vi "GetDeviceDetails.vi"(0 "reference in":refnum<class "Driver_Template.lvclass">, 11 "error in (no error)":errorcluster) -> (4 "reference out":refnum<class "Driver_Template.lvclass">, 6 "Name":string, 8 "Model":string, 10 "FW_Version":string, 13 "Is Device?":bool, 14 "SN":string, 15 "error out":errorcluster)   [LabVIEW 2014]
uses:
  Driver_Template.lvclass
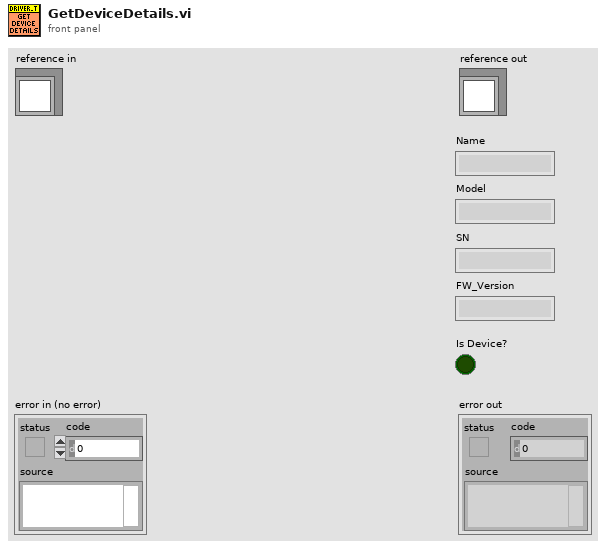
[diagram p1: front panel]
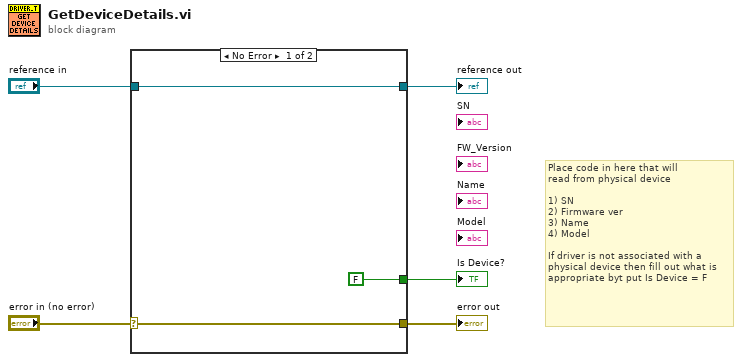
[diagram p0: block diagram]
diagram:
  # "Place code in here that will\nread from physical device\n\n1) SN\n2) Firmware ver\n3) Name\n4) Model\n\nIf driver is not associated with a\nphysical device then fill out what is\nappropriate byt put Is Device = F"
  n1 = case shown="No Error" "error in (no error)" {
    selector: "error in (no error)" -> [w7 w10]
    tunnel: [w7 w10] -> w4
    tunnel: [w6 w9] -> w2
    tunnel: "reference in" -> [w6 w9]
    tunnel: [FALSE ("Is Device?") _] -> w1
    frame No Error {
    }
    frame Error {
    }
  }
  "error out" <- w4
  "reference out" <- w2
  "Is Device?" <- w1
